vi "Read Name.vi"(8 "error in (no error)":errorcluster, 11 "Simulated Detector in":refnum<class "Simulated Detector.lvclass">) -> (0 "error out":errorcluster, 2 "Name":string, 3 "Simulated Detector out":refnum<class "Simulated Detector.lvclass">)   [LabVIEW 2019, in "Simulated Detector.lvclass"]
uses:
  Simulated Detector.lvclass
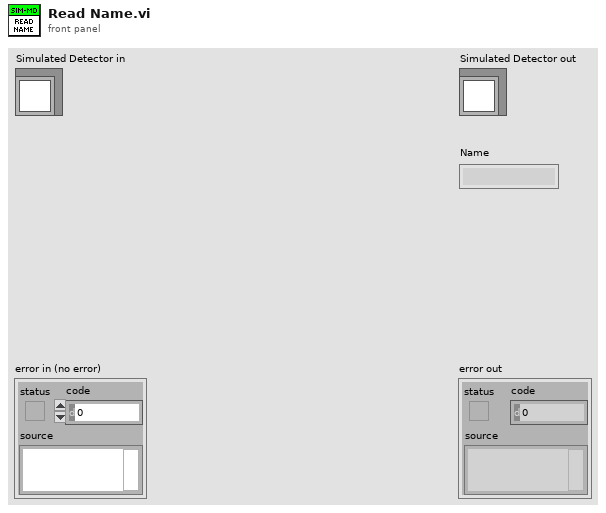
[diagram p1: front panel]
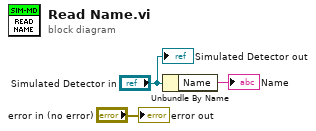
[diagram p0: block diagram]
diagram:
  n1 = Unbundle By Name("Simulated Detector in") -> ("Name"=→"Name":string)
  "error out" <- "error in (no error)"
  "Simulated Detector out" <- "Simulated Detector in"
